vi "TabControlStateMachine.vi"() -> ()   [LabVIEW 2010]
doc: "Use this template to build a standard state machine design pattern. Each state executes code and determines which state to transition to. Contrast this design pattern with the User Interface Event Handler pattern, in which code executes in response to user actions. Contrast this design pattern also with the Queued Message Handler pattern, in which each message handling code can queue zero or more new messages."
panel:
  in  "Boolean":bool
  in  "Tab Control":enum32{"Page 1", "Page 2"}(tab)
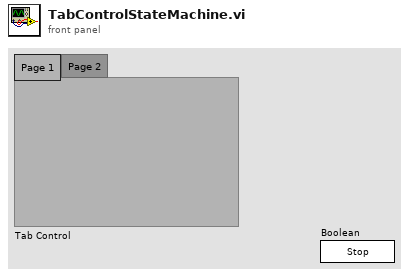
[diagram p1: front panel]
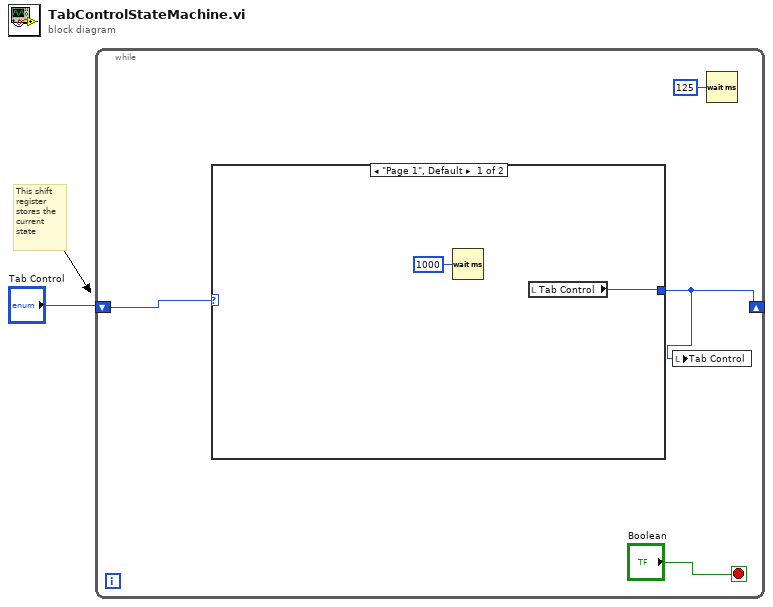
[diagram p0: block diagram]
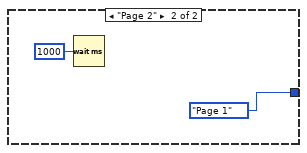
[diagram p2: hidden frame]
diagram:
  # "This shift\nregister\nstores the\ncurrent\nstate"
  n1 = while {
    shift-right: [w2] -> _
    shift-left: "Tab Control" -> [w4]
    stop <- "Boolean" stop-if-true
    n2 = case shown="\"Page 1\", Default" w4 {
      tunnel: [w6 enum32{"Page 1", "Page 2"}."Page 1" ("Tab Control")] -> w2
      frame "Page 1", Default {
        n3 = Wait (ms)(milliseconds to wait=u32 1000) -> ()  [unwired: 1 out]
        n4 = local read "Tab Control"() -> (w6:enum32{"Page 1", "Page 2"})
      }
      frame "Page 2" {
        n5 = Wait (ms)(milliseconds to wait=u32 1000) -> ()  [unwired: 1 out]
      }
    }
    n6 = local write "Tab Control"(w2) -> ()
    n7 = Wait (ms)(milliseconds to wait=u32 125) -> ()  [unwired: 1 out]
  }
